vi "Begin.vi"(8 "error in":errorcluster) -> (0 "error out":errorcluster)   [LabVIEW 2018]
doc: "Called before other user functions, this VI is expected to open initial I/O refnums, load in file data, and do all program initialization. Notice that the <B>error out</B> terminal is simply used for data flow. Wiring it to other structures or subVIs ensures that this VI runs first."
uses:
  <vilib>/Rock Robotics/WPI/Joystick/WPI_JoystickDeviceEnum.ctl
  <vilib>/Rock Robotics/SystemInterfaces/AI/FPGA_AIChannel.ctl
  <vilib>/Rock Robotics/WPI/Solenoid/WPI_SolenoidChannel.ctl
  <vilib>/Rock Robotics/SystemInterfaces/DIO/FPGA_DIORelayChannel.ctl
  <vilib>/Rock Robotics/WPI/Relay/WPI_RelayValue.ctl
  <vilib>/Rock Robotics/SystemInterfaces/DIO/FPGA_DIOPWMChannel.ctl
  <vilib>/Rock Robotics/SystemInterfaces/spilib/spi_bus.ctl
  <vilib>/Rock Robotics/SystemInterfaces/DIO/FPGA_DIOChannel.ctl
  <vilib>/Rock Robotics/WPI/Solenoid/WPI_SolenoidOpenSingle.vi
  <vilib>/Rock Robotics/WPI/Utilities/WPI_GetSetVariantRefNum.vi
  <vilib>/Rock Robotics/WPI/MotorControl/WPI_MotorControlOpen VictorSP.vi
  navx-mxp/labview/navX Library v2/IO/Open/Z900_navX_Open_SPI.vi
  <vilib>/Rock Robotics/WPI/Counter/WPI_CounterDigitalInputToDigitalSource.vi
  navx-mxp/labview/navX Library v2/navX Library v2.lvlib
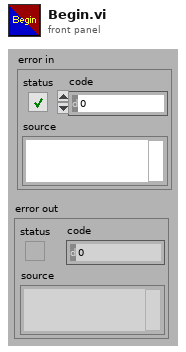
[diagram p1: front panel]
types:
  T1 = typedef "WPI_JoystickDeviceEnum.ctl" = enum16{"USB 0", "USB 1", "USB 2", "USB 3", "USB 4", "USB 5"}
  T2 = typedef "FPGA_AIChannel.ctl" = enum8{"AI 0", "AI 1", "AI 2", "AI 3", "AI MXP 0", "AI MXP 1", "AI MXP 2", "AI MXP 3", "Invalid"}
  T3 = typedef "FPGA_DIOPWMChannel.ctl" = enum8{"PWM 0", "PWM 1", "PWM 2", "PWM 3", "PWM 4", "PWM 5", "PWM 6", "PWM 7", "PWM 8", "PWM 9", "PWM MXP 0", "PWM MXP 1", "PWM MXP 2", "PWM MXP 3", "PWM MXP 4", "PWM MXP 5", "PWM MXP 6", "PWM MXP 7", "PWM MXP 8", "PWM MXP 9", "Invalid"}
  T4 = typedef "WPI_RelayValue.ctl" = enum16{"Off", "On", "Forward", "Reverse"}
  T5 = typedef "FPGA_DIORelayChannel.ctl" = enum8{"Relay 0", "Relay 1", "Relay 2", "Relay 3", "Invalid"}
  T6 = typedef "WPI_SolenoidChannel.ctl" = enum8{"Solenoid 0", "Solenoid 1", "Solenoid 2", "Solenoid 3", "Solenoid 4", "Solenoid 5", "Solenoid 6", "Solenoid 7", "Invalid"}
  T7 = typedef "spi_bus.ctl" = enum16{"SPI On-Board, CS0", "SPI On-Board, CS1", "SPI On-Board, CS2", "SPI On-Board, CS3", "SPI MXP", "Invalid"}
  T8 = typedef "WPI_JoystickDevRef.ctl" = cluster{"Device":T1}
  T9 = typedef "WPI_MotorControlDeviceRef.ctl" = cluster{"DeviceStatus":errorcluster, "Type":T10, "PWM":cluster{"PWM Channel":T3, "DeadBand":T11}, "CAN":cluster{"Device Number":u8, "SetOutput VI Ref":variant, "GetOutput VI Ref":variant, "Enable VI Ref":variant, "Disable VI Ref":variant, "Data":variant}, "Invert":bool, "DIO PWM":cluster{"PWM \"Enable\" Channel":T3, "DIOChannel":T12, "PWM Rate":dbl}}
  T10 = typedef "WPI_MotorControlType.ctl" = enum16{"PWM", "CAN", "DIO PWM"}
  T11 = typedef "WPI_PWMDeadband.ctl" = cluster{"Name":string, "maxPositivePwm":i32, "minPositivePwm":i32, "centerPwm":i32, "maxNegativePwm":i32, "minNegativePwm":i32, "angularRange":u16}
  T12 = typedef "FPGA_DIOChannel.ctl" = enum8{"DIO 0", "DIO 1", "DIO 2", "DIO 3", "DIO 4", "DIO 5", "DIO 6", "DIO 7", "DIO 8", "DIO 9", "DIO MXP 0", "DIO MXP 1", "DIO MXP 2", "DIO MXP 3", "DIO MXP 4", "DIO MXP 5", "DIO MXP 6", "DIO MXP 7", "DIO MXP 8", "DIO MXP 9", "DIO MXP 10", "DIO MXP 11", "DIO MXP 12", "DIO MXP 13", "DIO MXP 14", "DIO MXP 15", "SPI Port CS1", "SPI Port CS2", "SPI Port CS3", "SPI Port MISO", "SPI Port MOSI", "Invalid"}
  T13 = typedef "WPI_AnalogChannelDevRef.ctl" = cluster{"DevStatus":errorcluster, "Analog Channel":T2}
  T14 = typedef "WPI_CompressorDevRef.ctl" = cluster{"DevStatus":errorcluster, "Pneumatics Control Module":u8}
  T15 = typedef "WPI_RelayDevRef.ctl" = cluster{"DevStatus":errorcluster, "Relay Channel":T5, "Relay Direction":T16}
  T16 = typedef "WPI_RelayDirection.ctl" = enum16{"Both directions", "Forward only", "Reverse only"}
  T17 = typedef "WPI_SolenoidDevRef.ctl" = cluster{"DevStatus":errorcluster, "Pneumatics Control Module":u8, "Forward Solenoid Channel":T6, "Reverse Solenoid Channel":T6}
  T18 = typedef "navX Library v2.lvlib/Z900_navX_DeviceTypeDef.ctl" = cluster{"Interface":cluster{"Protocol":T19, "Update Rate (4Hz-100Hz)":u8, "navX Open TypeDef":variant}, "Notify Packet":refnum<notifier>, "Loop VI Refnum":refnum<vi>, "Ready to Close Occurrence Refnum":refnum<k4>}
  T19 = typedef "navX Library v2.lvlib/Z900_navX_ProtocolTypeDef.ctl" = enum16{"SERIAL", "I2C", "SPI"}
  T20 = typedef "WPI_DigitalInputDevRef.ctl" = cluster{"DevStatus":errorcluster, "DIO Channel":T12}
  T21 = typedef "FPGA_CounterEncoderSourceConvertionLVSourceType.ctl" = cluster{"DevStatus":errorcluster, "AnalogTriggerMode?":bool, "DigitalMode":cluster{"DIO Channel":T22}, "AnalogTriggerMode":cluster{"AnalogTriggerIndex":T23, "OutputType":T24}}
  T22 = typedef "FPGA_DIODigitalSourceChannel.ctl" = enum8{"DIO 0", "DIO 1", "DIO 2", "DIO 3", "DIO 4", "DIO 5", "DIO 6", "DIO 7", "DIO 8", "DIO 9", "DIO MXP 0", "DIO MXP 1", "DIO MXP 2", "DIO MXP 3", "DIO MXP 4", "DIO MXP 5", "DIO MXP 6", "DIO MXP 7", "DIO MXP 8", "DIO MXP 9", "DIO MXP 10", "DIO MXP 11", "DIO MXP 12", "DIO MXP 13", "DIO MXP 14", "DIO MXP 15", "SPI Port CS1", "SPI Port CS2", "SPI Port CS3", "SPI Port MISO", "SPI Port MOSI", "Disabled"}
  T23 = typedef "FPGA_AnalogTriggerIndex.ctl" = enum8{"Trig 0", "Trig 1", "Trig 2", "Trig 3", "Trig 4", "Trig 5", "Trig 6", "Trig 7", "Invalid"}
  T24 = typedef "FPGA_AnalogTriggerOutType.ctl" = enum16{"InWindow", "TriggerState", "Rising", "Falling"}
  T25 = typedef "WPI_EncoderDevRef.ctl" = cluster{"DevStatus":errorcluster, "EncoderIndex":T26, "CounterIndex":T27, "DistancePerCount":dbl, "Decoding Type":T28}
  T26 = typedef "FPGA_EncoderIdx.ctl" = enum8{"Enc 0", "Enc 1", "Enc 2", "Enc 3", "Enc 4", "Enc 5", "Enc 6", "Enc 7", "Invalid"}
  T27 = typedef "FPGA_CounterCtrSystemIndex.ctl" = enum8{"Ctr 0", "Ctr 1", "Ctr 2", "Ctr 3", "Ctr 4", "Ctr 5", "Ctr 6", "Ctr 7", "Invalid"}
  T28 = typedef "WPI_EncoderType.ctl" = enum16{"1x", "2x", "4x"}
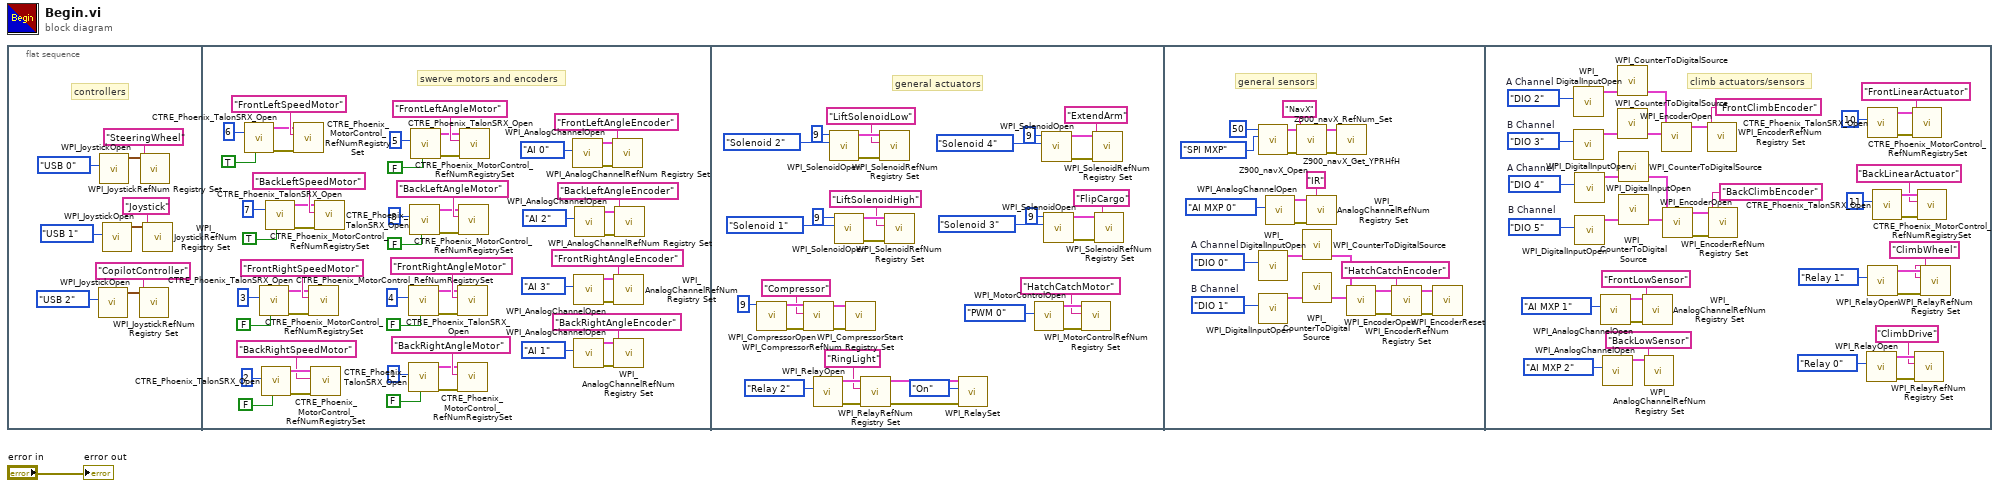
[diagram p0: block diagram]
diagram:
  n1 = flat-sequence {
    frame #0 {
      # "controllers"
      n2 = call <vilib>:"WPI_JoystickOpen.vi"("JoystickDevice"=WPI_JoystickDeviceEnum."USB 2") -> ("JoystickDevRef"=w4:T8)  [unwired: 10 in]
      n3 = call <vilib>:"WPI_JoystickOpen.vi"("JoystickDevice"=WPI_JoystickDeviceEnum."USB 0") -> ("JoystickDevRef"=w10:T8)  [unwired: 10 in]
      n4 = call <vilib>:"WPI_JoystickOpen.vi"("JoystickDevice"=WPI_JoystickDeviceEnum."USB 1") -> ("JoystickDevRef"=w7:T8)  [unwired: 10 in]
      n5 = call <vilib>:"WPI_JoystickRefNum Registry Set.vi"("refnum name"="CopilotController", "JoystickDevRef"=w4) -> ()  [unwired: 8 in, 2 out]
      n6 = call <vilib>:"WPI_JoystickRefNum Registry Set.vi"("refnum name"="SteeringWheel", "JoystickDevRef"=w10) -> ()  [unwired: 8 in, 2 out]
      n7 = call <vilib>:"WPI_JoystickRefNum Registry Set.vi"("refnum name"="Joystick", "JoystickDevRef"=w7) -> ()  [unwired: 8 in, 2 out]
    }
    frame #1 {
      # "swerve motors and encoders"
      n8 = call <vilib>:"CTRE_Phoenix_TalonSRX_Open.vi"("Invert"=TRUE, "Device Number"=u8 6) -> ("error out"=w52:errorcluster, "CAN Talon SRX Ref"=w53:T9)  [unwired: 8 in]
      n9 = call <vilib>:"CTRE_Phoenix_TalonSRX_Open.vi"("Invert"=FALSE, "Device Number"=u8 3) -> ("error out"=w56:errorcluster, "CAN Talon SRX Ref"=w57:T9)  [unwired: 8 in]
      n10 = call <vilib>:"CTRE_Phoenix_TalonSRX_Open.vi"("Invert"=FALSE, "Device Number"=u8 2) -> ("error out"=w58:errorcluster, "CAN Talon SRX Ref"=w59:T9)  [unwired: 8 in]
      n11 = call <vilib>:"CTRE_Phoenix_TalonSRX_Open.vi"("Invert"=TRUE, "Device Number"=u8 7) -> ("error out"=w54:errorcluster, "CAN Talon SRX Ref"=w55:T9)  [unwired: 8 in]
      n12 = call <vilib>:"CTRE_Phoenix_MotorControl_RefNumRegistrySet.vi"("error in (no error)"=w52, "refnum name"="FrontLeftSpeedMotor", "PhoenixMotorControlDevRef"=w53) -> ()  [unwired: 7 in, 2 out]
      n13 = call <vilib>:"CTRE_Phoenix_MotorControl_RefNumRegistrySet.vi"("error in (no error)"=w56, "refnum name"="FrontRightSpeedMotor", "PhoenixMotorControlDevRef"=w57) -> ()  [unwired: 7 in, 2 out]
      n14 = call <vilib>:"CTRE_Phoenix_MotorControl_RefNumRegistrySet.vi"("error in (no error)"=w58, "refnum name"="BackRightSpeedMotor", "PhoenixMotorControlDevRef"=w59) -> ()  [unwired: 7 in, 2 out]
      n15 = call <vilib>:"CTRE_Phoenix_MotorControl_RefNumRegistrySet.vi"("error in (no error)"=w54, "refnum name"="BackLeftSpeedMotor", "PhoenixMotorControlDevRef"=w55) -> ()  [unwired: 7 in, 2 out]
      n16 = call <vilib>:"CTRE_Phoenix_TalonSRX_Open.vi"("Invert"=FALSE, "Device Number"=u8 4) -> ("error out"=w38:errorcluster, "CAN Talon SRX Ref"=w39:T9)  [unwired: 8 in]
      n17 = call <vilib>:"CTRE_Phoenix_TalonSRX_Open.vi"("Invert"=FALSE, "Device Number"=u8 1) -> ("error out"=w36:errorcluster, "CAN Talon SRX Ref"=w37:T9)  [unwired: 8 in]
      n18 = call <vilib>:"CTRE_Phoenix_TalonSRX_Open.vi"("Invert"=FALSE, "Device Number"=u8 8) -> ("error out"=w40:errorcluster, "CAN Talon SRX Ref"=w41:T9)  [unwired: 8 in]
      n19 = call <vilib>:"CTRE_Phoenix_TalonSRX_Open.vi"("Invert"=FALSE, "Device Number"=u8 5) -> ("error out"=w42:errorcluster, "CAN Talon SRX Ref"=w43:T9)  [unwired: 8 in]
      n20 = call <vilib>:"CTRE_Phoenix_MotorControl_RefNumRegistrySet.vi"("error in (no error)"=w38, "refnum name"="FrontRightAngleMotor", "PhoenixMotorControlDevRef"=w39) -> ()  [unwired: 7 in, 2 out]
      n21 = call <vilib>:"CTRE_Phoenix_MotorControl_RefNumRegistrySet.vi"("error in (no error)"=w36, "refnum name"="BackRightAngleMotor", "PhoenixMotorControlDevRef"=w37) -> ()  [unwired: 7 in, 2 out]
      n22 = call <vilib>:"CTRE_Phoenix_MotorControl_RefNumRegistrySet.vi"("error in (no error)"=w40, "refnum name"="BackLeftAngleMotor", "PhoenixMotorControlDevRef"=w41) -> ()  [unwired: 7 in, 2 out]
      n23 = call <vilib>:"CTRE_Phoenix_MotorControl_RefNumRegistrySet.vi"("error in (no error)"=w42, "refnum name"="FrontLeftAngleMotor", "PhoenixMotorControlDevRef"=w43) -> ()  [unwired: 7 in, 2 out]
      n24 = call <vilib>:"WPI_AnalogChannelOpen.vi"("Analog Channel"=FPGA_AIChannel."AI 0") -> ("error out"=w34:errorcluster, "AIDeviceRef"=w35:T13)  [unwired: 9 in]
      n25 = call <vilib>:"WPI_AnalogChannelOpen.vi"("Analog Channel"=FPGA_AIChannel."AI 3") -> ("error out"=w26:errorcluster, "AIDeviceRef"=w27:T13)  [unwired: 9 in]
      n26 = call <vilib>:"WPI_AnalogChannelOpen.vi"("Analog Channel"=FPGA_AIChannel."AI 1") -> ("error out"=w22:errorcluster, "AIDeviceRef"=w23:T13)  [unwired: 9 in]
      n27 = call <vilib>:"WPI_AnalogChannelOpen.vi"("Analog Channel"=FPGA_AIChannel."AI 2") -> ("error out"=w30:errorcluster, "AIDeviceRef"=w31:T13)  [unwired: 9 in]
      n28 = call <vilib>:"WPI_AnalogChannelRefNum Registry Set.vi"("error in (no error)"=w34, "refnum name"="FrontLeftAngleEncoder", "AIDeviceRef"=w35) -> ()  [unwired: 7 in, 2 out]
      n29 = call <vilib>:"WPI_AnalogChannelRefNum Registry Set.vi"("error in (no error)"=w26, "refnum name"="FrontRightAngleEncoder", "AIDeviceRef"=w27) -> ()  [unwired: 7 in, 2 out]
      n30 = call <vilib>:"WPI_AnalogChannelRefNum Registry Set.vi"("error in (no error)"=w22, "refnum name"="BackRightAngleEncoder", "AIDeviceRef"=w23) -> ()  [unwired: 7 in, 2 out]
      n31 = call <vilib>:"WPI_AnalogChannelRefNum Registry Set.vi"("error in (no error)"=w30, "refnum name"="BackLeftAngleEncoder", "AIDeviceRef"=w31) -> ()  [unwired: 7 in, 2 out]
    }
    frame #2 {
      # "general actuators"
      n32 = call <vilib>:"WPI_CompressorOpen.vi"("Pneumatics Control Module (0)"=u8 9) -> ("CompressorDevRef"=w83:T14, "error out"=w82:errorcluster)  [unwired: 13 in]
      n33 = call <vilib>:"WPI_CompressorRefNum Registry Set.vi"("error in (no error)"=w82, "refnum name"="Compressor", "CompressorDevRef"=w83) -> ("error out"=w80:errorcluster, "CompressorDevRef"=w81:T14)  [unwired: 7 in]
      n34 = call <vilib>:"WPI_RelayOpen.vi"("Relay Channel"=FPGA_DIORelayChannel."Relay 2") -> ("error out"=w77:errorcluster, "RelayDevRef"=w76:T15)  [unwired: 9 in]
      n35 = call-poly <vilib>:"WPI_SolenoidOpen.vi"("Solenoid Channel"=WPI_SolenoidChannel."Solenoid 2", "Pneumatics Control Module (0)"=u8 9) -> ("error out"=w94:errorcluster, "SolenoidDevRef"=w103:T17)  [unwired: 8 in]
      n36 = call-poly <vilib>:"WPI_SolenoidOpen.vi"("Solenoid Channel"=WPI_SolenoidChannel."Solenoid 1", "Pneumatics Control Module (0)"=u8 9) -> ("error out"=w95:errorcluster, "SolenoidDevRef"=w101:T17)  [unwired: 8 in]
      n37 = call <vilib>:"WPI_CompressorStart.vi"("error in (no error)"=w80, "CompressorDevRef"=w81) -> ()  [unwired: 8 in, 2 out]
      n38 = call <vilib>:"WPI_RelayRefNum Registry Set.vi"("error in (no error)"=w77, "refnum name"="RingLight", "RelayDevRef"=w76) -> ("error out"=w74:errorcluster, "RelayDevRef"=w75:T15)  [unwired: 7 in]
      n39 = call <vilib>:"WPI_SolenoidRefNum Registry Set.vi"("error in (no error)"=w94, "refnum name"="LiftSolenoidLow", "SolenoidDevRef"=w103) -> ()  [unwired: 7 in, 2 out]
      n40 = call <vilib>:"WPI_SolenoidRefNum Registry Set.vi"("error in (no error)"=w95, "refnum name"="LiftSolenoidHigh", "SolenoidDevRef"=w101) -> ()  [unwired: 7 in, 2 out]
      n41 = call <vilib>:"WPI_RelaySet.vi"("error in (no error)"=w74, "RelayValue"=WPI_RelayValue."On", "RelayDevRef"=w75) -> ()  [unwired: 7 in, 2 out]
      n42 = call-poly <vilib>:"WPI_MotorControlOpen.vi"("PWM Channel"=FPGA_DIOPWMChannel."PWM 0") -> ("error out"=w70:errorcluster, "MotorControlDeviceRef"=w69:T9)  [unwired: 9 in]
      n43 = call-poly <vilib>:"WPI_SolenoidOpen.vi"("Solenoid Channel"=WPI_SolenoidChannel."Solenoid 4", "Pneumatics Control Module (0)"=u8 9) -> ("error out"=w89:errorcluster, "SolenoidDevRef"=w93:T17)  [unwired: 8 in]
      n44 = call-poly <vilib>:"WPI_SolenoidOpen.vi"("Solenoid Channel"=WPI_SolenoidChannel."Solenoid 3", "Pneumatics Control Module (0)"=u8 9) -> ("error out"=w84:errorcluster, "SolenoidDevRef"=w88:T17)  [unwired: 8 in]
      n45 = call <vilib>:"WPI_MotorControlRefNum Registry Set.vi"("error in (no error)"=w70, "refnum name"="HatchCatchMotor", "MotorControlDevRef"=w69) -> ()  [unwired: 7 in, 2 out]
      n46 = call <vilib>:"WPI_SolenoidRefNum Registry Set.vi"("error in (no error)"=w89, "refnum name"="ExtendArm", "SolenoidDevRef"=w93) -> ()  [unwired: 7 in, 2 out]
      n47 = call <vilib>:"WPI_SolenoidRefNum Registry Set.vi"("error in (no error)"=w84, "refnum name"="FlipCargo", "SolenoidDevRef"=w88) -> ()  [unwired: 7 in, 2 out]
    }
    frame #3 {
      w114 = FPGA_DIOChannel."DIO 1"  # B Channel
      w113 = FPGA_DIOChannel."DIO 0"  # A Channel
      # "general sensors"
      n48 = call-poly "Z900_navX_Open.vi"("SPI Bus"=spi_bus."SPI MXP", "Update Rate (4Hz-60Hz)"=u8 50) -> ("error out"=w125:errorcluster, "navX Device"=w124:T18)  [unwired: 8 in]
      n49 = call <vilib>:"WPI_DigitalInputOpen.vi"("DIO Channel"=w113) -> ("DigitalInputDevRef"=w110:T20)  [unwired: 1 in, 9 out]
      n50 = call <vilib>:"WPI_DigitalInputOpen.vi"("DIO Channel"=w114) -> ("DigitalInputDevRef"=w111:T20)  [unwired: 1 in, 9 out]
      n51 = call <vilib>:"WPI_AnalogChannelOpen.vi"("Analog Channel"=FPGA_AIChannel."AI MXP 0") -> ("error out"=w117:errorcluster, "AIDeviceRef"=w118:T13)  [unwired: 9 in]
      n52 = call "Z900_navX_RefNum_Set.vi"("error in (no error)"=w125, "refnum name"="NavX", "navX Device"=w124) -> ("error out"=w120:errorcluster, "navX Device"=w121:T18)  [unwired: 7 in]
      n53 = call-poly <vilib>:"WPI_CounterToDigitalSource.vi"("DigitalInputDevRef"=w110) -> ("Digital Source"=w109:T21)  [unwired: 6 out]
      n54 = call-poly <vilib>:"WPI_CounterToDigitalSource.vi"("DigitalInputDevRef"=w111) -> ("Digital Source"=w112:T21)  [unwired: 6 out]
      n55 = call <vilib>:"WPI_AnalogChannelRefNum Registry Set.vi"("error in (no error)"=w117, "refnum name"="IR", "AIDeviceRef"=w118) -> ()  [unwired: 7 in, 2 out]
      n56 = call "Z900_navX_Get_YPRHfH.vi"("error in (no error)"=w120, "navX Device"=w121) -> ()  [unwired: 6 in, 4 out]
      n57 = call <vilib>:"WPI_EncoderOpen.vi"("BSource"=w112, "ASource"=w109) -> ("error out"=w108:errorcluster, "EncoderDevRef"=w107:T25)  [unwired: 6 in, 2 out]
      n58 = call <vilib>:"WPI_EncoderRefNum Registry Set.vi"("error in (no error)"=w108, "refnum name"="HatchCatchEncoder", "EncoderDevRef"=w107) -> ("error out"=w105:errorcluster, "EncoderDevRef"=w104:T25)  [unwired: 7 in]
      n59 = call <vilib>:"WPI_EncoderReset.vi"("error in (no error)"=w105, "EncoderDevRef"=w104) -> ()  [unwired: 8 in, 2 out]
    }
    frame #4 {
      w150 = FPGA_DIOChannel."DIO 5"  # B Channel
      w149 = FPGA_DIOChannel."DIO 4"  # A Channel
      w159 = FPGA_DIOChannel."DIO 3"  # B Channel
      w158 = FPGA_DIOChannel."DIO 2"  # A Channel
      # "climb actuators/sensors"
      n60 = call <vilib>:"WPI_DigitalInputOpen.vi"("DIO Channel"=w158) -> ("DigitalInputDevRef"=w163:T20)  [unwired: 1 in, 9 out]
      n61 = call <vilib>:"WPI_DigitalInputOpen.vi"("DIO Channel"=w159) -> ("DigitalInputDevRef"=w164:T20)  [unwired: 1 in, 9 out]
      n62 = call <vilib>:"WPI_DigitalInputOpen.vi"("DIO Channel"=w149) -> ("DigitalInputDevRef"=w154:T20)  [unwired: 1 in, 9 out]
      n63 = call <vilib>:"WPI_DigitalInputOpen.vi"("DIO Channel"=w150) -> ("DigitalInputDevRef"=w153:T20)  [unwired: 1 in, 9 out]
      n64 = call <vilib>:"WPI_AnalogChannelOpen.vi"("Analog Channel"=FPGA_AIChannel."AI MXP 1") -> ("error out"=w135:errorcluster, "AIDeviceRef"=w136:T13)  [unwired: 9 in]
      n65 = call <vilib>:"WPI_AnalogChannelOpen.vi"("Analog Channel"=FPGA_AIChannel."AI MXP 2") -> ("AIDeviceRef"=w132:T13)  [unwired: 9 in, 1 out]
      n66 = call-poly <vilib>:"WPI_CounterToDigitalSource.vi"("DigitalInputDevRef"=w163) -> ("Digital Source"=w162:T21)  [unwired: 6 out]
      n67 = call-poly <vilib>:"WPI_CounterToDigitalSource.vi"("DigitalInputDevRef"=w164) -> ("Digital Source"=w165:T21)  [unwired: 6 out]
      n68 = call-poly <vilib>:"WPI_CounterToDigitalSource.vi"("DigitalInputDevRef"=w154) -> ("Digital Source"=w155:T21)  [unwired: 6 out]
      n69 = call-poly <vilib>:"WPI_CounterToDigitalSource.vi"("DigitalInputDevRef"=w153) -> ("Digital Source"=w152:T21)  [unwired: 6 out]
      n70 = call <vilib>:"WPI_AnalogChannelRefNum Registry Set.vi"("error in (no error)"=w135, "refnum name"="FrontLowSensor", "AIDeviceRef"=w136) -> ()  [unwired: 7 in, 2 out]
      n71 = call <vilib>:"WPI_AnalogChannelRefNum Registry Set.vi"("refnum name"="BackLowSensor", "AIDeviceRef"=w132) -> ()  [unwired: 8 in, 2 out]
      n72 = call <vilib>:"WPI_EncoderOpen.vi"("BSource"=w165, "ASource"=w162) -> ("EncoderDevRef"=w161:T25)  [unwired: 6 in, 3 out]
      n73 = call <vilib>:"WPI_EncoderOpen.vi"("BSource"=w152, "ASource"=w155) -> ("error out"=w156:errorcluster, "EncoderDevRef"=w157:T25)  [unwired: 6 in, 2 out]
      n74 = call <vilib>:"WPI_EncoderRefNum Registry Set.vi"("refnum name"="FrontClimbEncoder", "EncoderDevRef"=w161) -> ()  [unwired: 8 in, 2 out]
      n75 = call <vilib>:"WPI_EncoderRefNum Registry Set.vi"("error in (no error)"=w156, "refnum name"="BackClimbEncoder", "EncoderDevRef"=w157) -> ()  [unwired: 7 in, 2 out]
      n76 = call <vilib>:"WPI_RelayOpen.vi"("Relay Channel"=FPGA_DIORelayChannel."Relay 0") -> ("error out"=w140:errorcluster, "RelayDevRef"=w138:T15)  [unwired: 9 in]
      n77 = call <vilib>:"CTRE_Phoenix_TalonSRX_Open.vi"("Device Number"=u8 10) -> ("error out"=w148:errorcluster, "CAN Talon SRX Ref"=w147:T9)  [unwired: 9 in]
      n78 = call <vilib>:"WPI_RelayOpen.vi"("Relay Channel"=FPGA_DIORelayChannel."Relay 1") -> ("error out"=w129:errorcluster, "RelayDevRef"=w128:T15)  [unwired: 9 in]
      n79 = call <vilib>:"CTRE_Phoenix_TalonSRX_Open.vi"("Device Number"=u8 11) -> ("error out"=w144:errorcluster, "CAN Talon SRX Ref"=w143:T9)  [unwired: 9 in]
      n80 = call <vilib>:"CTRE_Phoenix_MotorControl_RefNumRegistrySet.vi"("error in (no error)"=w148, "refnum name"="FrontLinearActuator", "PhoenixMotorControlDevRef"=w147) -> ()  [unwired: 7 in, 2 out]
      n81 = call <vilib>:"WPI_RelayRefNum Registry Set.vi"("error in (no error)"=w140, "refnum name"="ClimbDrive", "RelayDevRef"=w138) -> ()  [unwired: 7 in, 2 out]
      n82 = call <vilib>:"CTRE_Phoenix_MotorControl_RefNumRegistrySet.vi"("error in (no error)"=w144, "refnum name"="BackLinearActuator", "PhoenixMotorControlDevRef"=w143) -> ()  [unwired: 7 in, 2 out]
      n83 = call <vilib>:"WPI_RelayRefNum Registry Set.vi"("error in (no error)"=w129, "refnum name"="ClimbWheel", "RelayDevRef"=w128) -> ()  [unwired: 7 in, 2 out]
    }
  }
  "error out" <- "error in"
